vi "Receive (ErrorIn and ObsReg).vi"(7 "ObserverRegistry in":refnum<class "ObserverRegistry.lvclass">, 8 "error in (no error)":errorcluster, 9 "timeout in ms (-1)":i32=5000, 11 "MGR in":refnum<class "MGR (Receive type).lvclass">) -> (0 "error out":errorcluster, 1 "Label":string, 2 "Message":refnum<class "MSG.lvclass">, 3 "MGR out":refnum<class "MGR (Receive type).lvclass">)   [LabVIEW 2011, in "Messenging.lvlib" / "MGR (Receive type).lvclass"]
uses:
  MGR (Receive type).lvclass
  ErrorMessage/ErrorMessage.lvclass
  TextVarientMessage/MSG.lvclass
  Parallel Process/ObserverRegister/ObserverRegistry.lvclass
panel:
  # "MSRReceiveTimedOut"
  # "MSRReceiverError"
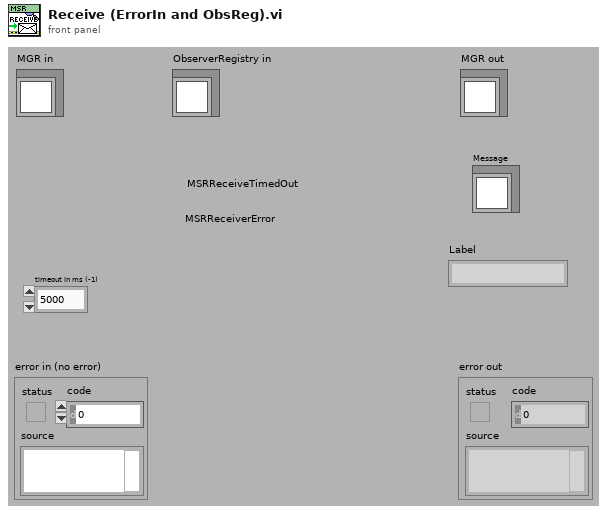
[diagram p1: front panel]
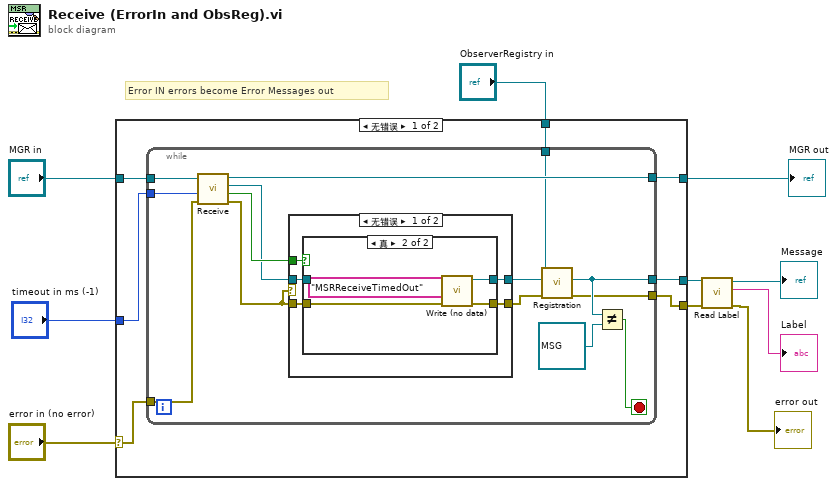
[diagram p0: block diagram]
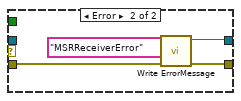
[diagram p3: hidden frame]
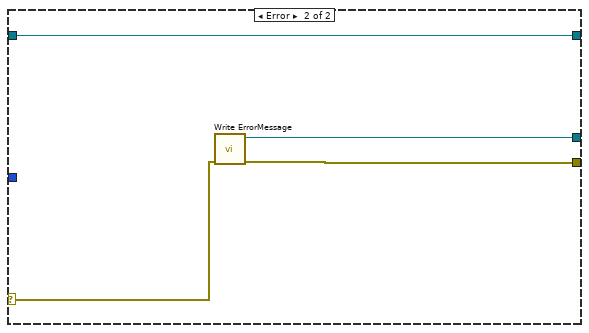
[diagram p4: hidden frame]
diagram:
  # "Error IN errors become Error Messages out"
  n1 = case shown="无错误" "error in (no error)" {
    selector: "error in (no error)" -> [w14 w47]
    tunnel: [w11 w48] -> w3
    tunnel: [w16 w50] -> w8
    tunnel: "MGR in" -> [w17 w50]
    tunnel: "timeout in ms (-1)" -> [w15 _]
    tunnel: [w12 w49] -> w6
    tunnel: "ObserverRegistry in" -> [w13 _]
    frame No Error {
      n2 = while {
        tunnel: w17 -> [w31]
        tunnel: [w30] -> w16
        tunnel: w15 -> [w29]
        tunnel: w14 -> [w28]
        tunnel: w13 -> [w23]
        tunnel: [w21] -> w12
        tunnel: [w18] -> w11
        stop <- w19 stop-if-true
        n3 = call-dynamic "Receive.vi"("error in (no error)"=w28, "timeout in ms (-1)"=w29, "Messenger in"=w31) -> ("error out"=w25:errorcluster, "timed out?"=w27:bool, "Message"=w26:refnum<class "MSG.lvclass">, "Messenger out"=w30:refnum<class "MGR (Receive type).lvclass">)  [unwired: 5 out]
        n4 = case shown="无错误" w25 {
          tunnel: w27 -> [w36 _]
          tunnel: w26 -> [w35 _]
          tunnel: w25 -> [w34 w44]
          tunnel: [w33 w45] -> w24
          tunnel: [w32 w46] -> w22
          frame No Error {
            n5 = case shown="真" w36 {
              tunnel: [w38 w41] -> w33
              tunnel: w35 -> [w38 _]
              tunnel: w34 -> [w37 w40]
              tunnel: [w37 w39] -> w32
              frame False {
              }
              frame True {
                n6 = call "Write (no data).vi"("error in (no error)"=w40, "Label"="MSRReceiveTimedOut" ("Text")) -> ("error out"=w39:errorcluster, "Message"=w41:refnum<class "MSG.lvclass">)  [unwired: 8 out]
              }
            }
          }
          frame Error {
            n7 = call "Write ErrorMessage.vi"("error (to be sent)"=w44, "Label"="MSRReceiverError") -> ("error out"=w46:errorcluster, "Message"=w45:refnum<class "ErrorMessage.lvclass">)  [unwired: 1 in, 7 out]
          }
        }
        n8 = call "Registration.vi"("error in (no error)"=w22, "Message"=w24, "ObserverRegistry in"=w23) -> ("error out"=w18:errorcluster, "Message (Register Commands filtered out)"=w21:refnum<class "MSG.lvclass">)  [unwired: 7 out]
        n9 = Not Equal?(x=w21, y=refnum<class "MSG.lvclass"> refnum ("Messenging.lvlib:Interprocess Message")) -> (x != y?=w19:bool)
      }
    }
    frame Error {
      n10 = call "Write ErrorMessage.vi"("error (to be sent)"=w47) -> ("error out"=w48:errorcluster, "Message"=w49:refnum<class "ErrorMessage.lvclass">)  [unwired: 2 in, 7 out]
    }
  }
  "MGR out" <- w8
  n11 = call-dynamic "Read Label.vi"("error in (no error)"=w3, "Message"=w6) -> ("error out"=→"error out":errorcluster, "Label"=→"Label":string, "Message"=→"Message":refnum<class "MSG.lvclass">)  [unwired: 7 out]
